vi "Remove repeat item names.vi"(11 "names":string[](array[string])) -> (3 "Array":string[](array[string]))   [LabVIEW 2018]
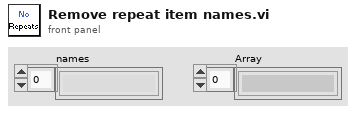
[diagram p1: front panel]
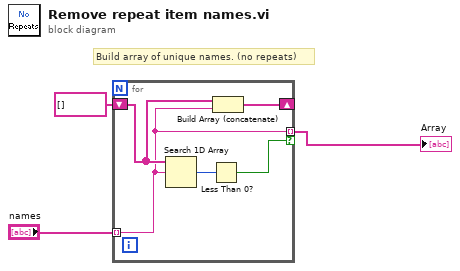
[diagram p0: block diagram]
diagram:
  # "Build array of unique names. (no repeats)"
  n1 = for {
    tunnel: "names" -> [w5] mode=indexing
    tunnel: [w5] -> w3 mode=indexing if=w7
    shift-right: [w6] -> _
    shift-left: string[] [] ("names") -> [w8]
    n2 = Search 1D Array(1D array=w8, element=w5) -> (index of element=w4:i32)  [unwired: 1 in]
    n3 = Less Than 0?(x=w4) -> (x < 0?=w7:bool)
    n4 = Build Array (concatenate)(w8, w5) -> (w6:string[])
  }
  "Array" <- w3
